vi "New Terminal Reference Binding.vi"(9 "Signaling Write? (T)":bool=TRUE, 10 "Ctl Refnum":refnum<vi>) -> (0 "error out":errorcluster, 3 "TerminalReference out":refnum<class "TerminalReference.lvclass">)   [LabVIEW 2015, in "Mediator.lvlib" / "TerminalReference.lvclass"]
doc: "<License>\nCopyright © 2017 Composed Systems, LLC | All rights reserved\nwww.composed.io\n\nAuthor: Ethan Stern <ethan.stern@composed.io>\n\nThis software is provided \"AS IS\" WITHOUT WARRANTIES, either express or implied, AND IS FOR EDUCATIONAL PURPOSES ONLY.\n</License>"
uses:
  TerminalReference.lvclass
  TerminalReference.lvclass/TerminalReference.ctl
panel:
  # "If you don't need Value(Sgnl) writes, use the\nTerminalBinding transport type--it is much faster."
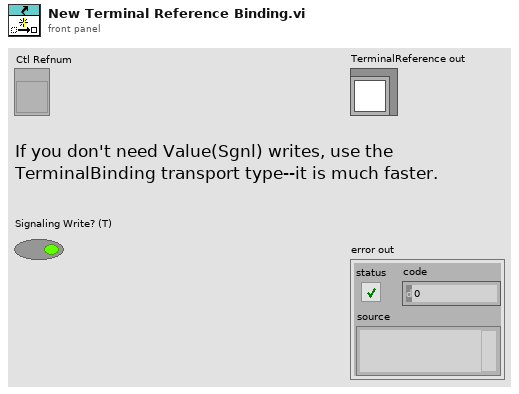
[diagram p1: front panel]
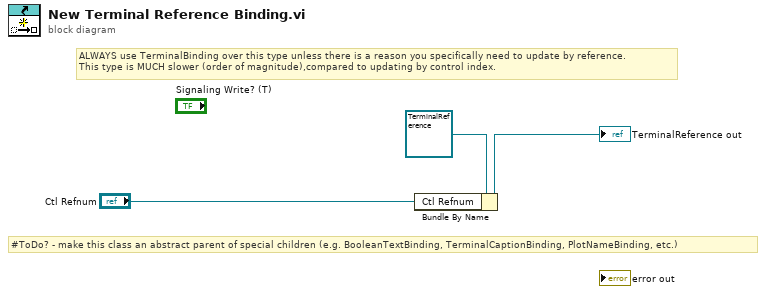
[diagram p0: block diagram]
diagram:
  # "#ToDo? - make this class an abstract parent of special children (e.g. BooleanTextBinding, TerminalCaptionBinding, PlotNameBinding, etc.)"
  # "ALWAYS use TerminalBinding over this type unless there is a reason you specifically need to update by reference.\nThis type is MUCH slower (order of magnitude),compared to updating by control index."
  n1 = Bundle By Name(cluster=refnum<class "TerminalReference.lvclass"> refnum ("TerminalReference in"), "Ctl Refnum"="Ctl Refnum") -> (→"TerminalReference out":refnum<class "TerminalReference.lvclass">)
